vi "Kill Kitty.vi"(8 "error in (no error)":errorcluster caption="entrée d'erreur (pas d'erreur)") -> (0 "error out":errorcluster caption="sortie d'erreur")   [LabVIEW 2020, in "Library Test.lvlib" / "P2265_SwitchOn_Test.lvclass"]
uses:
  P2265_SwitchOn_Test.lvclass
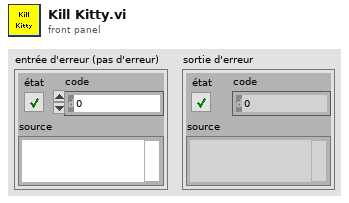
[diagram p1: front panel]
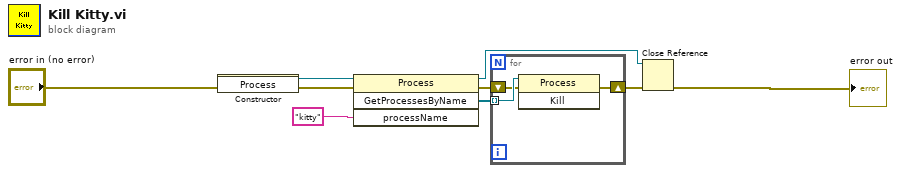
[diagram p0: block diagram]
diagram:
  n1 = constructor class="Process"(error in="error in (no error)") -> (reference out=w9:refnum<k24>, error out=w6:errorcluster)  [unwired: 2 in, 1 out]
  n2 = invoke class="Process" method="GetProcessesByName"(reference=w9, error in=w6, "processName"="kitty") -> (reference out=w3:refnum<k24>, error out=w5:errorcluster, "GetProcessesByName"=w7:refnum<k24>[])  [unwired: 1 in, 1 out]
  n3 = for {
    tunnel: w7 -> [w12] mode=indexing
    shift-right: [w10] -> w4
    shift-left: w5 -> [w11]
    n4 = invoke class="Process" method="Kill"(reference=w12, error in=w11) -> (error out=w10:errorcluster)  [unwired: 1 in, 2 out]
  }
  n5 = Close Reference(reference=w3, error in (no error)=w4) -> (error out=→"error out":errorcluster)
